vi "FitToDrawArea__slk_mt.vi"(8 "error in (no error)":errorcluster, 10 "total bounds":T1, 11 "view in":refnum<class "View__slk_mt.lvclass">) -> (0 "error out":errorcluster, 3 "view out":refnum<class "View__slk_mt.lvclass">)   [LabVIEW 2010, in "Lazyboots Menu Tool.lvlib" / "View__slk_mt.lvclass"]
doc: "Scales to fit draw area of view object."
uses:
  View__slk_mt.lvclass
  <vilib>/Utility/miscctls.llb/LVRectTypeDef.ctl
  View__slk_mt.lvclass/View__slk_mt.ctl
panel:
  # "FitToDrawArea__slk_mt.vi\nScales to fit draw area of view object.\n\nNOTICE -- YOU MUST LEAVE THIS NOTICE IN PLACE.\n\nCopyright (c) 2011, LIANG LIU Shawn.Liu.cn@gmail.com\nAll rights reserved.\n\nRedistribution and use in source and binary forms, with or without modification, are permitted provided that the following conditions are met:\n-Redistributions of source code must retain the above copyright notice, this list of conditions and the following disclaimer.\n-Redistributions in binary form must reproduce the above copyright notice, this list of conditions and the following disclaimer in the documentation and/or other materials provided with the distribution.\n-Neither the name of the eLp nor the names of its contributors may be used to endorse or promote products derived from this software without specific prior written permission.\n\nTHIS SOFTWARE IS PROVIDED BY THE COPYRIGHT HOLDERS AND CONTRIBUTORS \"AS IS\" AND ANY EXPRESS OR IMPLIED WARRANTIES, INCLUDING, BUT NOT LIMITED TO, THE IMPLIED WARRANTIES OF MERCHANTABILITY AND FITNESS FOR A PARTICULAR PURPOSE ARE DISCLAIMED. IN NO EVENT SHALL THE COPYRIGHT HOLDER OR CONTRIBUTORS BE LIABLE FOR ANY DIRECT, INDIRECT, INCIDENTAL, SPECIAL, EXEMPLARY, OR CONSEQUENTIAL DAMAGES (INCLUDING, BUT NOT LIMITED TO, PROCUREMENT OF SUBSTITUTE GOODS OR SERVICES; LOSS OF USE, DATA, OR PROFITS; OR BUSINESS INTERRUPTION) HOWEVER CAUSED AND ON ANY THEORY OF LIABILITY, WHETHER IN CONTRACT, STRICT LIABILITY, OR TORT (INCLUDING NEGLIGENCE OR OTHERWISE) ARISING IN ANY WAY OUT OF THE USE OF THIS SOFTWARE, EVEN IF ADVISED OF THE POSSIBILITY OF SUCH DAMAGE."
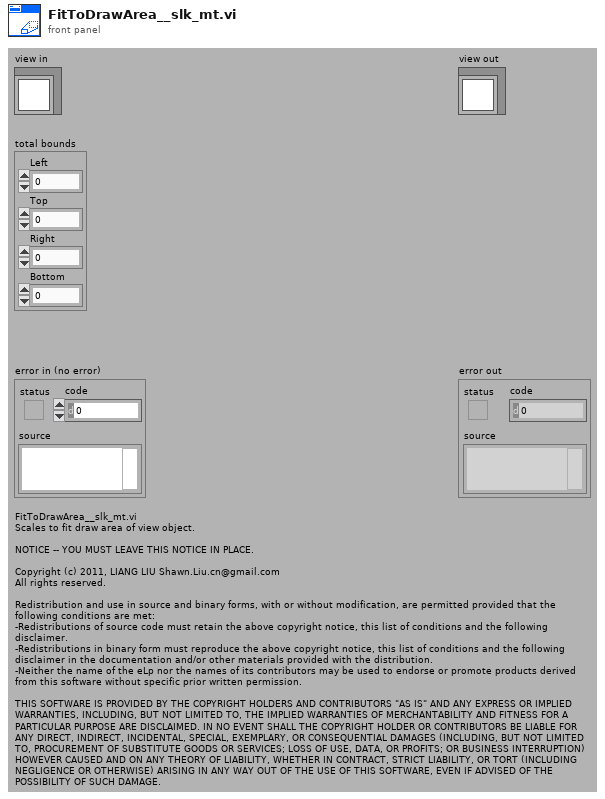
[diagram p1: front panel]
types:
  T1 = typedef "LVRectTypeDef.ctl" = cluster{"Left":i16, "Top":i16, "Right":i16, "Bottom":i16}
  T2 = typedef "LVBoundsTypeDef.ctl" = cluster{"Width":u32, "Height":u32}
  T3 = typedef "LVPointTypeDef.ctl" = cluster{"Horizontal":i16, "Vertical":i16}
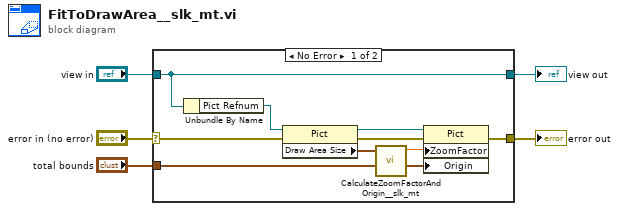
[diagram p0: block diagram]
diagram:
  n1 = case shown="No Error" "error in (no error)" {
    selector: "error in (no error)" -> [w8 w17]
    tunnel: [w11 w17] -> w4
    tunnel: [w15 w16] -> w2
    tunnel: "view in" -> [w15 w16]
    tunnel: "total bounds" -> [w7 _]
    frame No Error {
      n2 = Unbundle By Name(w15) -> ("Pict Refnum"=w14:refnum<vi>)
      n3 = property class="Pict"(reference=w14, error in=w8) -> (reference out=w13:refnum<vi>, error out=w12:errorcluster, "Draw Area Size"=w10:T2)
      n4 = call "CalculateZoomFactorAndOrigin__slk_mt.vi"("bounds rectangle"=w7, "draw area size"=w10) -> ("origin"=w9:T3, "zoom factor"=w6:dbl)  [unwired: 8 in]
      n5 = property class="Pict"(reference=w13, error in=w12, "ZoomFactor"=w6, "Origin"=w9) -> (error out=w11:errorcluster)  [unwired: 1 out]
    }
    frame Error {
    }
  }
  "error out" <- w4
  "view out" <- w2
